vi "Work.vi"(0 "Action":T4=enum."Start", 1 "Init":T3 {"Numeric" format="%.3p"}, 2 "Tag":T2 {"Numeric" format="%.3p"}, 5 "In":dbl format="%.3p", 12 "State in":T1 {"Numeric" format="%.3p"}) -> (3 "No Output":bool, 4 "Out":dbl format="%.3p", 14 "State out":T1 {"Numeric" format="%.3p"}, 15 "Error":errorcluster)   [LabVIEW 2020, in "Worker Template.lvlib"]
uses:
  Worker Template.lvlib
  Worker Action.ctl
  FlexBlocks.lvlib
  Init.ctl
  Tag.ctl
  State.ctl
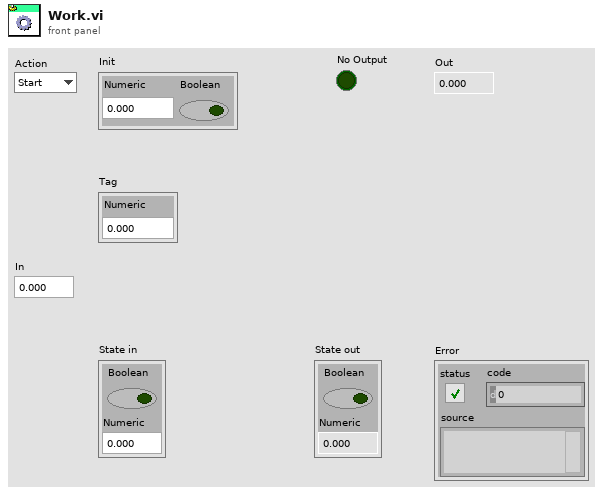
[diagram p1: front panel]
types:
  T1 = typedef "Worker Template.lvlib/State.ctl" = cluster{"Boolean":bool, "Numeric":dbl}
  T2 = typedef "Worker Template.lvlib/Tag.ctl" = cluster{"Numeric":dbl}
  T3 = typedef "Worker Template.lvlib/Init.ctl" = cluster{"Numeric":dbl, "Boolean":bool}
  T4 = typedef "FlexBlocks.lvlib/Worker Action.ctl" = enum16{"Init", "Start", "Work", "Stop", "Close"}
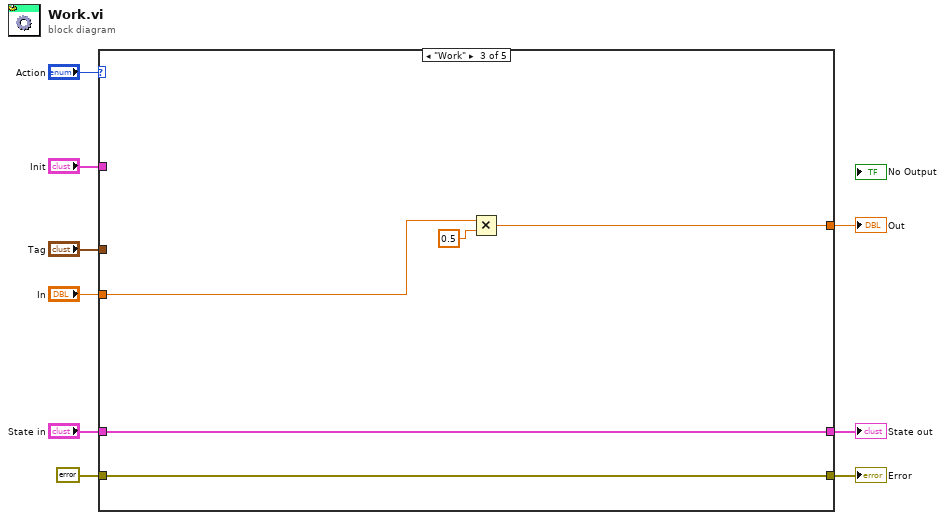
[diagram p0: block diagram]
diagram:
  n1 = case shown="\"Work\"" "Action" {
    tunnel: "State in" -> [w11 w13 w18 w20 w22]
    tunnel: [w11 w13 w18 w20 w22] -> w7
    tunnel: "Init" -> [_ _ _ _ _]
    tunnel: "Tag" -> [_ _ _ _ _]
    tunnel: "In" -> [_ _ w17 _ _]
    tunnel: errorcluster {"status"=FALSE, "code"=0, "source"=""} ("error constant") -> [w10 w12 w15 w19 w21]
    tunnel: [w10 w12 w15 w19 w21] -> w2
    tunnel: [_ _ w16 _ _] -> w1
    frame "Init" {
    }
    frame "Start" {
    }
    frame "Work" {
      n2 = Multiply(x=w17, y=0.5) -> (x*y=w16:dbl)
    }
    frame "Stop" {
    }
    frame "Close" {
    }
  }
  "State out" <- w7
  "Error" <- w2
  "Out" <- w1
